vi "save data.vi"(7 "experiment name":string="01_90_01", 8 "samples":cdb[](array[numeric]), 9 "csi":cdb[](array[numeric]), 10 "?":bool=TRUE, 11 "packet number":u32=30) -> (0 "error out":errorcluster, 1 "Done":bool=TRUE, 2 "packet number in buf":u32=30, 3 "packets in buf (%)":dbl(slide)=1000.0 scale=0.0..1.0, 4 "samples string buffer":string, 6 "csi string buffer":string)   [LabVIEW 2020]
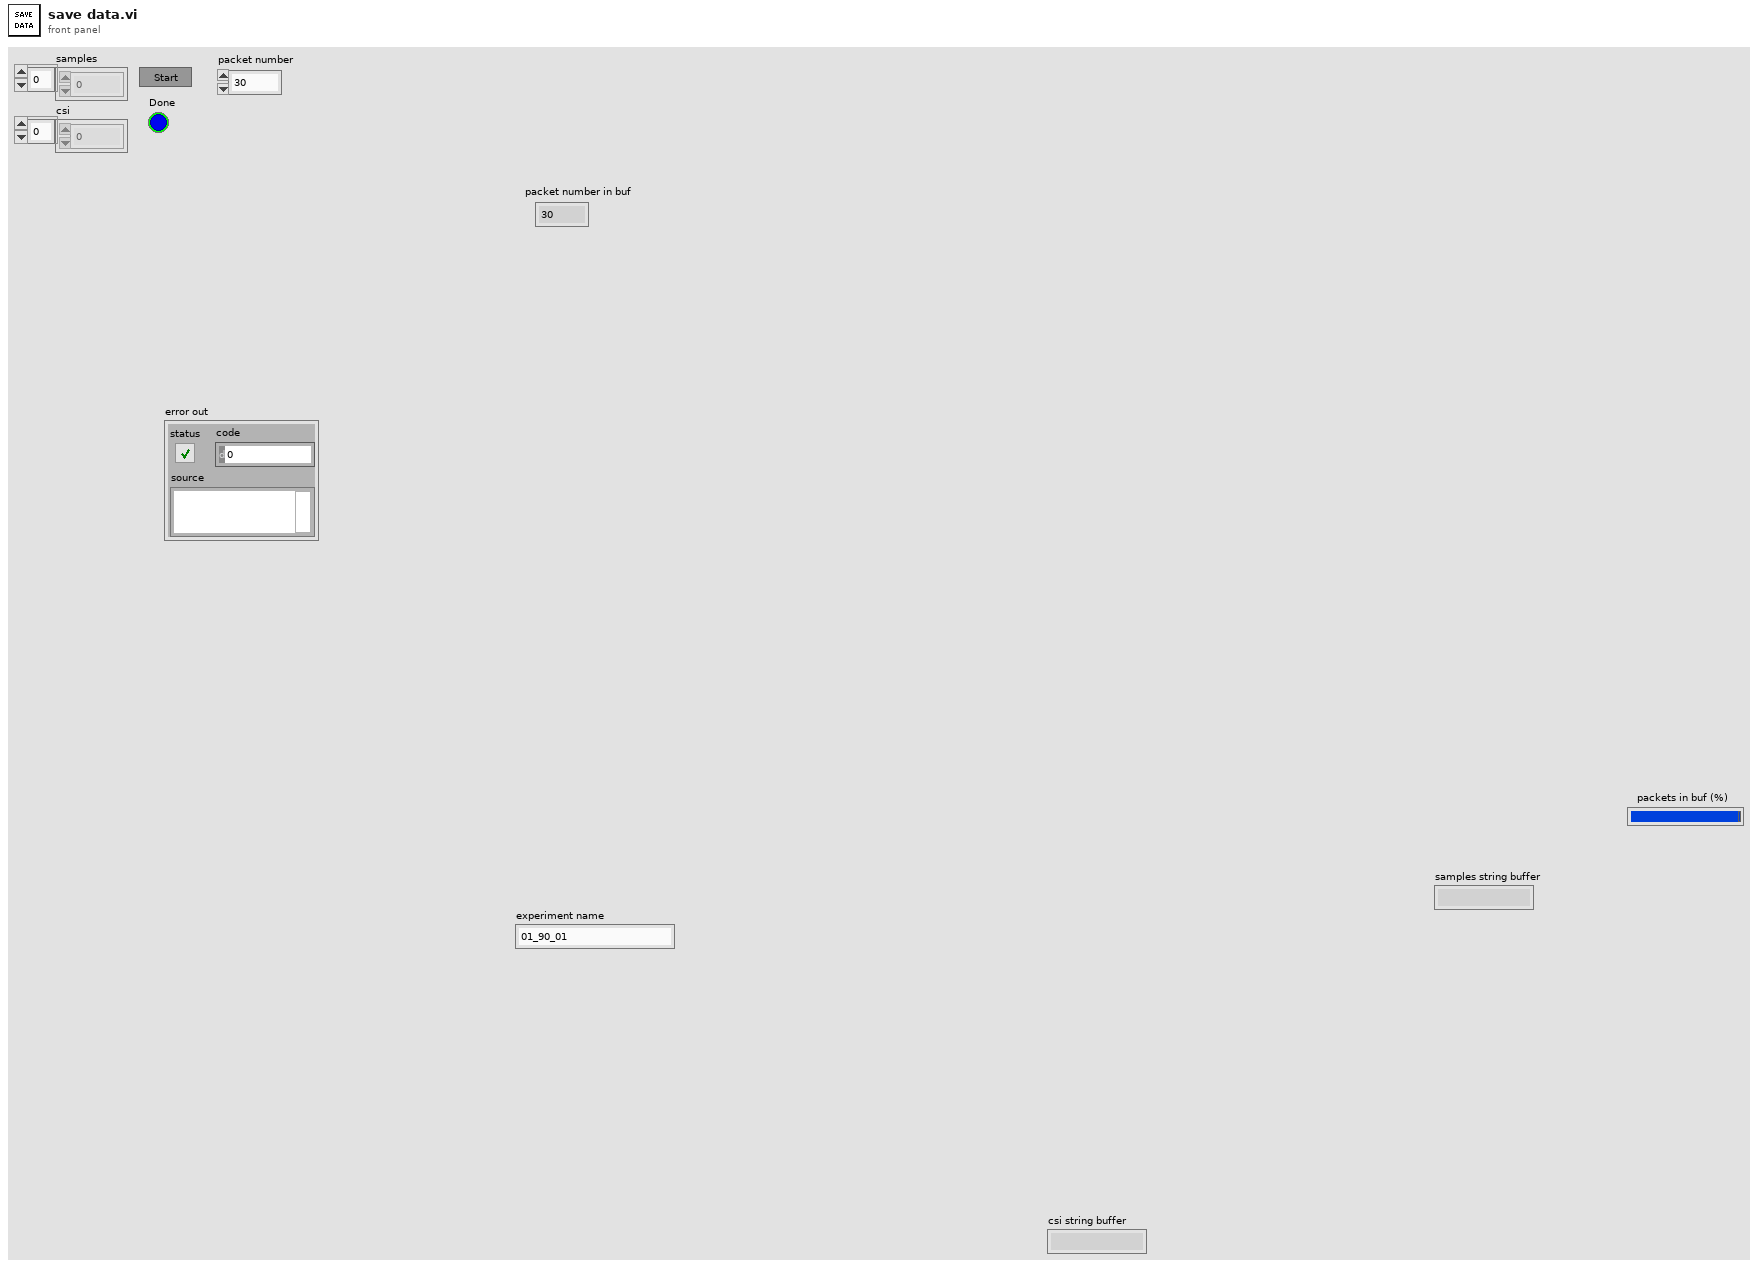
[diagram p1: front panel]
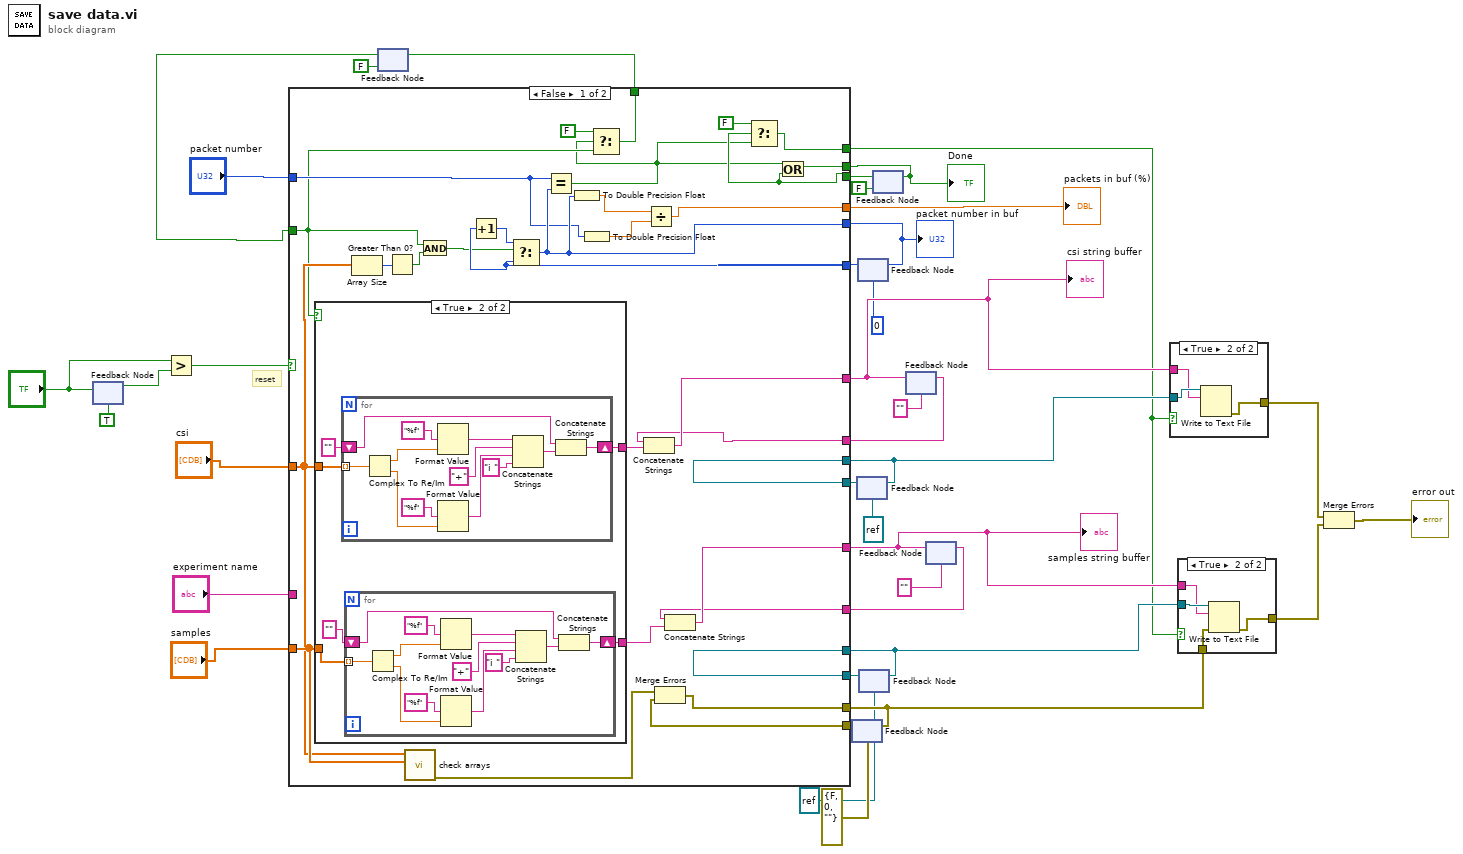
[diagram p0: block diagram]
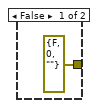
[diagram p3: hidden frame]
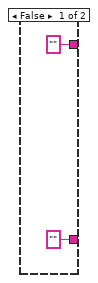
[diagram p4: hidden frame]
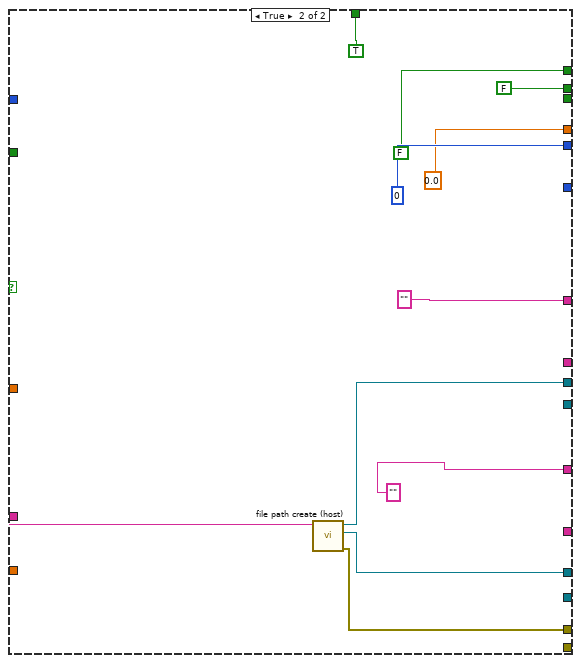
[diagram p5: hidden frame]
diagram:
  # "reset"
  n1 = feedback #1(TRUE) -> (w36:bool)
  n2 = feedback-in #1("?") -> ()
  n3 = Greater?(x="?", y=w36) -> (0:w33:bool)
  n4 = feedback #2(FALSE ("t")) -> (w9:bool)
  n5 = feedback #3(errorcluster {"status"=FALSE, "code"=0, "source"=""} ("error out")) -> (w22:errorcluster)
  n6 = feedback #4(refnum<file> refnum ("csi file")) -> (w23:refnum<file>)
  n7 = feedback #5(u32 0 ("packet number in buf")) -> (w17:u32)
  n8 = feedback #6(refnum<file> refnum ("samples file")) -> (w25:refnum<file>)
  n9 = feedback #7(FALSE) -> (w8:bool)
  n10 = feedback #8("" ("output string")) -> (w14:string)
  n11 = feedback #9("" ("output string")) -> (w12:string)
  n12 = case shown="False" w33 {
    tunnel: "experiment name" -> [_ w111]
    tunnel: [w55 ""] -> w29
    tunnel: [w66 w109] -> w24
    tunnel: [w65 w108] -> w26
    tunnel: w25 -> [w65 _]
    tunnel: w23 -> [w66 _]
    tunnel: [w63 w107] -> w21
    tunnel: w22 -> [w64 _]
    tunnel: "samples" -> [w50 _]
    tunnel: "csi" -> [w48 _]
    tunnel: [w57 u32 0 ("packet number in buf")] -> w18
    tunnel: w9 -> [w44 _]
    tunnel: w17 -> [w61 _]
    tunnel: "packet number" -> [w56 _]
    tunnel: [w39 FALSE] -> w11
    tunnel: [w58 0.0] -> w15
    tunnel: w14 -> [w54 _]
    tunnel: [w53 ""] -> w13
    tunnel: w12 -> [w52 _]
    tunnel: [w45 TRUE] -> w10
    tunnel: [w42 FALSE] -> w7
    tunnel: w8 -> [w41 _]
    frame False {
      n13 = case shown="True" w44 {
        tunnel: ["" w74] -> w68
        tunnel: ["" w73] -> w67
        tunnel: w50 -> [_ w72]
        tunnel: w48 -> [_ w71]
        frame False {
        }
        frame True {
          n14 = for {
            shift-right: [w99] -> w73
            shift-left: "" -> [w100]
            tunnel: w71 -> [w89] mode=indexing
            n15 = Complex To Re/Im(x + iy=w89) -> (x=w91:dbl, y=w90:dbl)
            n16 = Format Value(format string="%f", value (0)=w91) -> (output string=w98:string)  [unwired: 1 in]
            n17 = Format Value(format string="%f", value (0)=w90) -> (output string=w97:string)  [unwired: 1 in]
            n18 = Concatenate Strings(w98, "+" ("string"), w97, "i " ("string")) -> (w92:string)
            n19 = Concatenate Strings(w100, w92) -> (w99:string)
          }
          n20 = for {
            shift-right: [w87] -> w74
            shift-left: "" -> [w88]
            tunnel: w72 -> [w77] mode=indexing
            n21 = Complex To Re/Im(x + iy=w77) -> (x=w79:dbl, y=w78:dbl)
            n22 = Format Value(format string="%f", value (0)=w79) -> (output string=w86:string)  [unwired: 1 in]
            n23 = Format Value(format string="%f", value (0)=w78) -> (output string=w85:string)  [unwired: 1 in]
            n24 = Concatenate Strings(w86, "+" ("string"), w85, "i " ("string")) -> (w80:string)
            n25 = Concatenate Strings(w88, w80) -> (w87:string)
          }
        }
      }
      n26 = Array Size(array=w48) -> (size(s)=w49:i32)
      n27 = Greater Than 0?(x=w49) -> (x > 0?=w47:bool)
      n28 = call "check arrays.vi"("array 2"=w50, "array 1"=w48) -> ("error out"=w51:errorcluster)  [unwired: 9 in]
      n29 = And(x=w44, y=w47) -> (x .and. y?=w46:bool)
      n30 = Increment(x=w61) -> (x+1=w62:u32)
      n31 = Select(t=w62, s=w46, f=w61) -> (s? t:f=w57:u32)
      n32 = Equal?(x=w56, y=w57) -> (x = y?=w40:bool)
      n33 = To Double Precision Float(number=w57) -> (double precision float=w60:dbl)
      n34 = To Double Precision Float(number=w56) -> (double precision float=w59:dbl)
      n35 = Select(t=FALSE, s=w40, f=w44) -> (s? t:f=w45:bool)
      n36 = Concatenate Strings(w54, w67) -> (w55:string)
      n37 = Divide(x=w60, y=w59) -> (x/y=w58:dbl)
      n38 = Merge Errors(w51, w64) -> (w63:errorcluster)
      n39 = Concatenate Strings(w52, w68) -> (w53:string)
      n40 = Select(t=FALSE, s=w41, f=w40) -> (s? t:f=w39:bool)
      n41 = Or(x=w40, y=w41) -> (x .or. y?=w42:bool)
    }
    frame True {
      n42 = call "file path create (host).vi"("experiment name"=w111) -> ("error out"=w107:errorcluster, "samples file"=w108:refnum<file>, "csi file"=w109:refnum<file>)  [unwired: 8 in]
    }
  }
  "Done" <- w7
  "samples string buffer" <- w13
  "csi string buffer" <- w29
  "packet number in buf" <- w18
  "packets in buf (%)" <- w15
  n43 = feedback-in #2(w10) -> ()
  n44 = feedback-in #3(w21) -> ()
  n45 = feedback-in #4(w24) -> ()
  n46 = feedback-in #5(w18) -> ()
  n47 = feedback-in #6(w26) -> ()
  n48 = feedback-in #7(w7) -> ()
  n49 = feedback-in #8(w29) -> ()
  n50 = feedback-in #9(w13) -> ()
  n51 = case shown="True" w11 {
    tunnel: w24 -> [_ w115]
    tunnel: w29 -> [_ w114]
    tunnel: [errorcluster {"status"=FALSE, "code"=0, "source"=""} ("error out") w113] -> w28
    frame False {
    }
    frame True {
      n52 = Write to Text File(file (use dialog)=w115, text=w114) -> (error out=w113:errorcluster)  [unwired: 2 in, 2 out]
    }
  }
  n53 = case shown="True" w11 {
    tunnel: w26 -> [_ w120]
    tunnel: w13 -> [_ w119]
    tunnel: [w116 w118] -> w27
    tunnel: w21 -> [w116 w117]
    frame False {
    }
    frame True {
      n54 = Write to Text File(file (use dialog)=w120, text=w119, error in=w117) -> (error out=w118:errorcluster)  [unwired: 1 in, 2 out]
    }
  }
  n55 = Merge Errors(w28, w27) -> (→"error out":errorcluster)
